vi "File Append.vi"() -> ()   [LabVIEW 2026]
panel:
  in  "file path":path
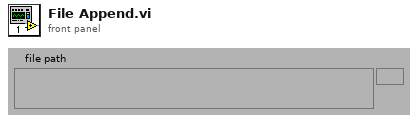
[diagram p1: front panel]
types:
  T1 = enum16{"open", "open or create", "create or replace", "create", "open (read only)"}
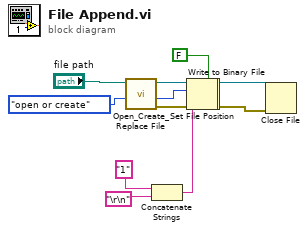
[diagram p0: block diagram]
diagram:
  n1 = call <vilib>:"Open_Create_Replace File.vi"("function (open:0)"=T1."open or create", "file path"="file path") -> ("error out"=w11:errorcluster, "file size (bytes)"=w9:i32, "refnum"=w10:refnum<file>)  [unwired: 6 in, 1 out]
  n2 = Concatenate Strings("1", "\r\n") -> (w4:string)
  n3 = Set File Position(offset (in bytes) (0)=w9, refnum=w10, error in=w11) -> (refnum out=w3:refnum<file>, error out=w2:errorcluster)  [unwired: 1 in]
  n4 = Write to Binary File(file (use dialog)=w3, data=w4, error in=w2, 5:FALSE ("prepend array or string size? (T)")) -> (refnum out=w7:refnum<file>, error out=w8:errorcluster)  [unwired: 2 in, 1 out]
  n5 = Close File(refnum=w7, error in=w8) -> ()  [unwired: 2 out]
